vi "Queue Nested.vi"(8 "Alias":string, 9 "Priority?":bool, 10 "Msg Strategy":refnum<class "Msg Strategy.lvclass">, 11 "Hello World Queue in":refnum<class "Hello World Queue.lvclass">) -> (3 "Hello World Queue out":refnum<class "Hello World Queue.lvclass">)   [LabVIEW 2021, in "Hello World Queue.lvlib" / "Hello World Queue.lvclass"]
uses:
  Hello World Queue.lvclass
  jettl/Msg Strategy/Msg Strategy.lvclass
  Hello World Queue.lvclass/Hello World Queue.ctl
  jettl/jettl/Queue jettl/Queue jettl.lvclass
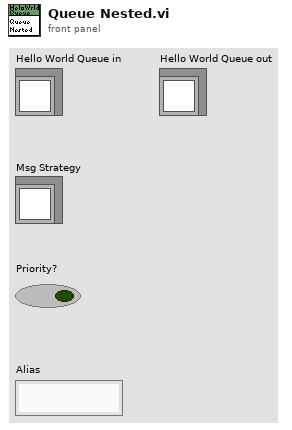
[diagram p1: front panel]
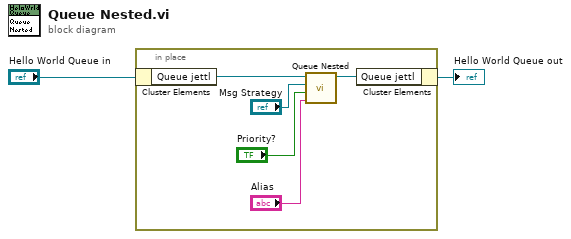
[diagram p0: block diagram]
diagram:
  n1 = in-place {
    n2 = in-place-cluster #1("Hello World Queue in") -> ("Queue jettl"=w7:refnum<class "Queue jettl.lvclass">)
    n3 = call-dynamic "Queue Nested.vi"("Alias"="Alias", "Priority?"="Priority?", "Msg Strategy"="Msg Strategy", "jettl in"=w7) -> ("jettl out"=w6:refnum<class "Queue jettl.lvclass">)  [unwired: 7 in]
    n4 = in-place-cluster #1("Queue jettl"=w6) -> (→"Hello World Queue out":refnum<class "Hello World Queue.lvclass">)
  }
